vi "Transmitter_Example_Image.vi"() -> ()   [LabVIEW 2018]
uses:
  <vilib>/picture/picture.llb/imagedata.ctl
  <instrlib>/niUSRP/niUSRP Write Tx Data (CDB Cluster).vi
panel:
  out "bits":i32[](array[numeric])
  out "new picture":picture
  out "image data":T1
  in  "path to BMP file":path
  in  "Modulation parameter":T2
  out "Bits length":i32
  out "Frame Duration":dbl format="%#_6p"
  out "Waveform Graph":cluster{"t0":dbl, "dt":dbl, "Y":dbl[]}(graph)
  in  "stop":bool
  out "USRP CoercedParamters":T3={"coerced IQ rate"=100000.0, "coerced carrier frequency"=100000.0, "coerced gain"=0.0} {"coerced gain" format="%#_6f"; "coerced carrier frequency" format="%#_6p"; "coerced IQ rate" format="%#_6p"}
  out "error out":errorcluster
  in  "error in (no error)":errorcluster
  in  "USRP ControledParameters":T4={"active antenna"="TX1", "gain"=0.0, "carrier frequency"=915000000.0, "IQ rate"=1000000.0} {"IQ rate" format="%#_6p"; "carrier frequency" format="%#_6p"; "gain" format="%#_6f"}
  in  "device names":refnum<k15>="192.168.10.1"
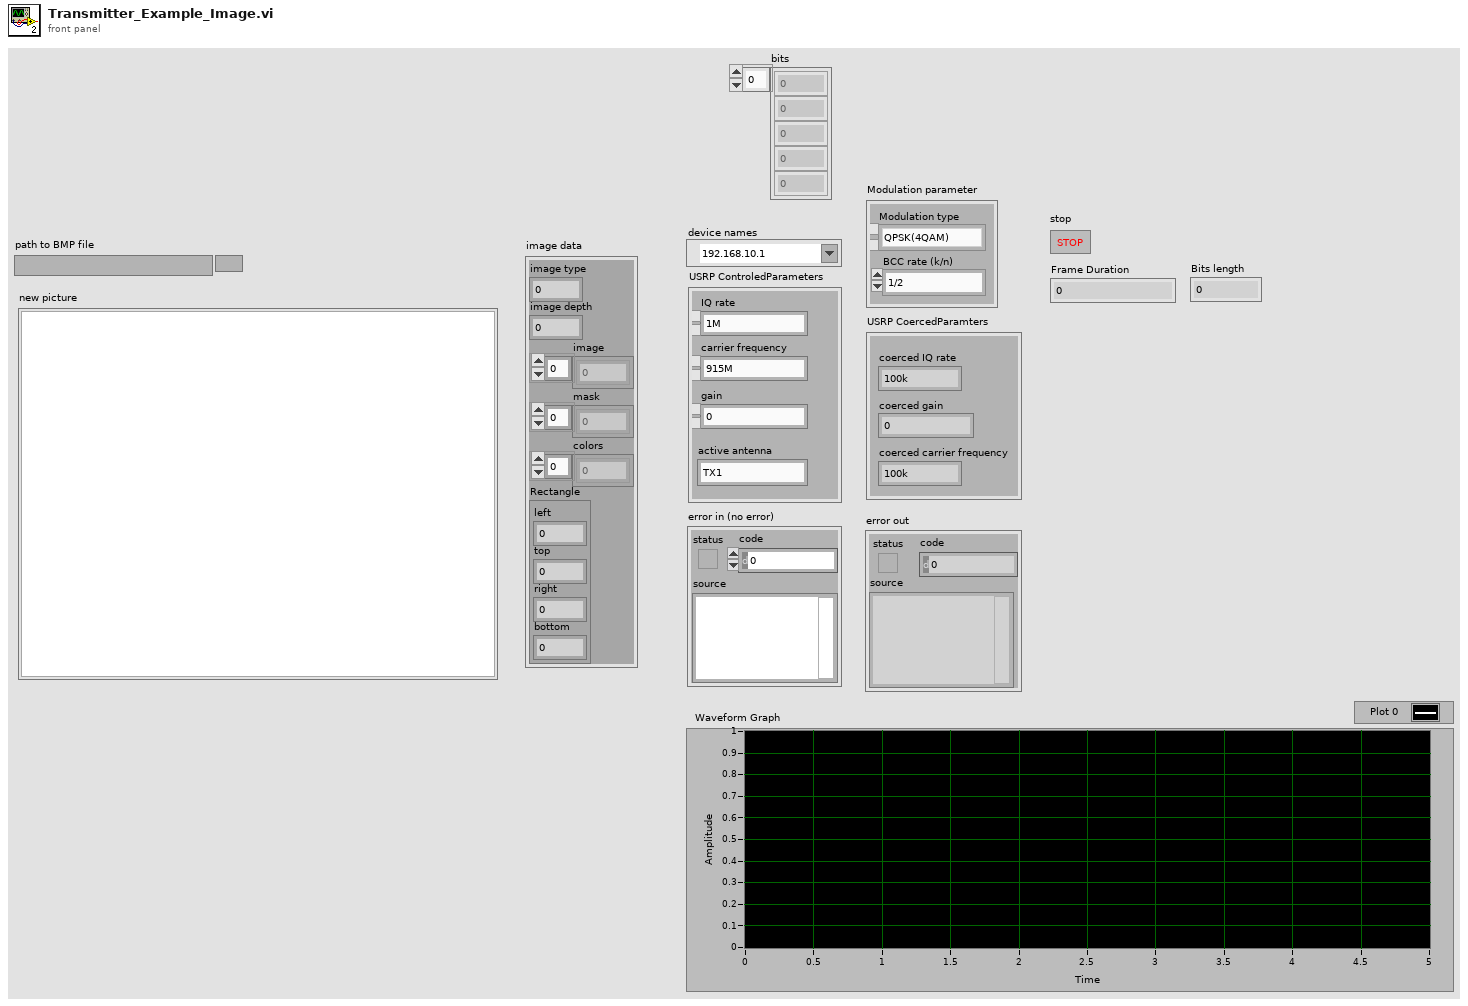
[diagram p1: front panel]
types:
  T1 = typedef "imagedata.ctl" = cluster{"image type":i32, "image depth":i32, "image":u8[], "mask":u8[], "colors":u32[], "Rectangle":cluster{"left":i16, "top":i16, "right":i16, "bottom":i16}}
  T2 = cluster{"Modulation type":enum16{"QPSK(4QAM)", "64QAM", "16QAM", "BPSK"}, "BCC rate (k/n)":enum16{"1/2", "2/3", "3/4"}}
  T3 = cluster{"coerced IQ rate":dbl, "coerced carrier frequency":dbl, "coerced gain":dbl}
  T4 = cluster{"active antenna":string, "gain":dbl, "carrier frequency":dbl, "IQ rate":dbl}
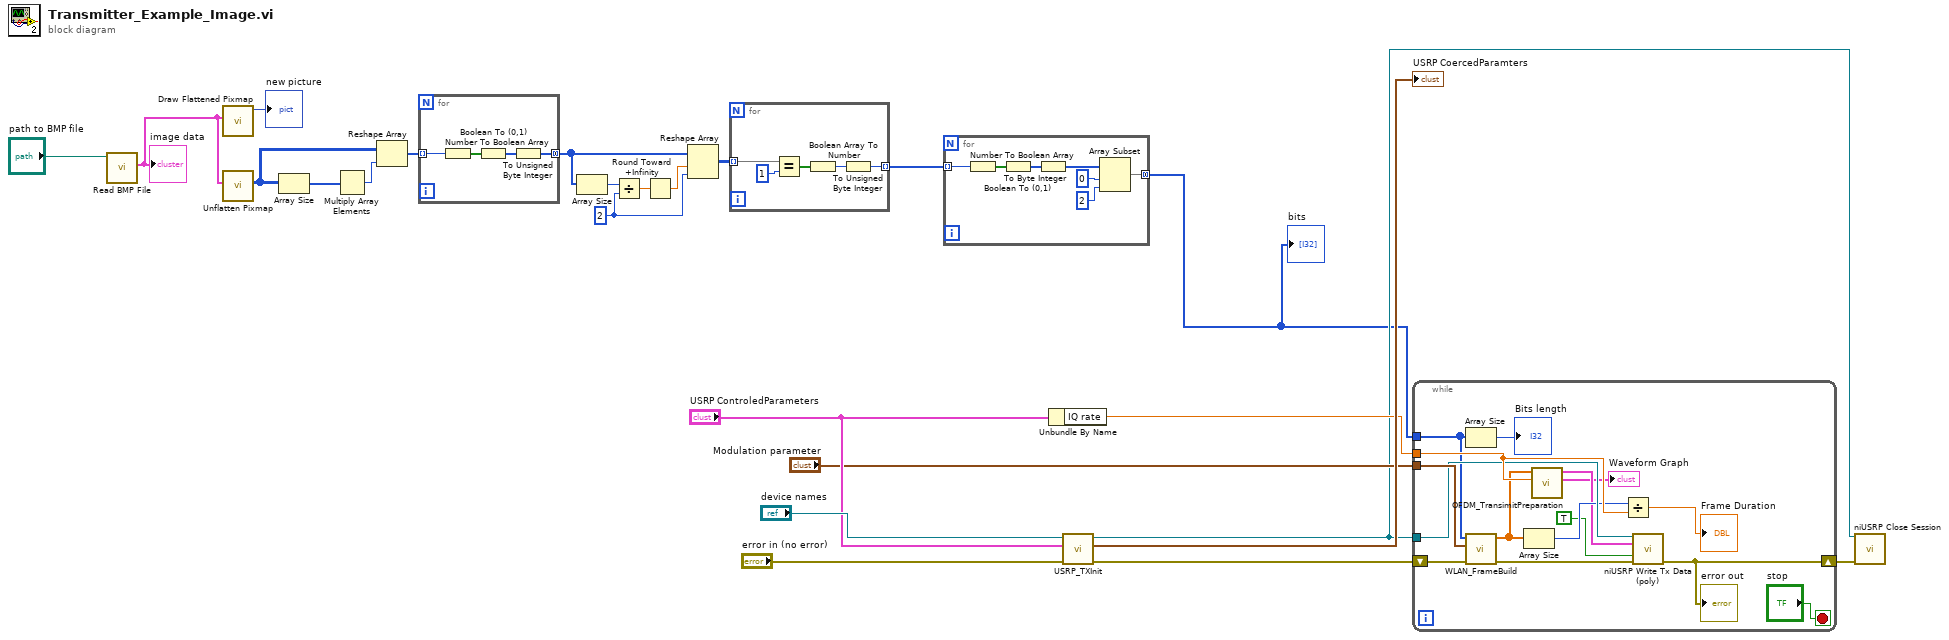
[diagram p0: block diagram]
diagram:
  w8 = 2 ("y")
  n1 = call <vilib>:"Read BMP File.vi"("path to BMP file"="path to BMP file") -> ("image data"=w13:T1)  [unwired: 8 in, 2 out]
  "image data" <- w13
  n2 = call <vilib>:"Draw Flattened Pixmap.vi"("image data"=w13) -> ("new picture"=→"new picture":picture)  [unwired: 8 in]
  n3 = call <vilib>:"Unflatten Pixmap.vi"("image data"=w13) -> ("8-bit pixmap"=w10:u8[][])  [unwired: 4 in, 6 out]
  n4 = Array Size(array=w10) -> (size(s)=w12:i32[])
  n5 = Multiply Array Elements(1:w12) -> (0:w11:i32)
  n6 = Reshape Array(w10, w11) -> (w9:u8[])
  n7 = for {
    tunnel: w9 -> [w27] mode=indexing
    tunnel: [w25] -> w4 mode=concatenating
    n8 = Number To Boolean Array(number=w27) -> (Boolean array=w28:bool[])
    n9 = Boolean To (0,1)(Boolean=w28) -> (0, 1=w26:i16[])
    n10 = To Unsigned Byte Integer(number=w26) -> (unsigned 8bit integer=w25:u8[])
  }
  n11 = Array Size(array=w4) -> (size(s)=w5:i32)
  n12 = Divide(x=w5, y=w8) -> (x/y=w6:dbl)
  n13 = Round Toward +Infinity(x=w6) -> (ceil(x): smallest int >= x=w7:dbl)
  n14 = Reshape Array(w4, w7, w8) -> (w3:u8[][])
  n15 = for {
    tunnel: w3 -> [w30] mode=indexing
    tunnel: [w29] -> w2 mode=indexing
    n16 = Equal?(x=w30, y=1) -> (x = y?=w32:bool[])
    n17 = Boolean Array To Number(Boolean array=w32) -> (number=w31:u32)
    n18 = To Unsigned Byte Integer(number=w31) -> (unsigned 8bit integer=w29:u8)
  }
  n19 = for {
    tunnel: w2 -> [w40] mode=indexing
    tunnel: [w34] -> w1 mode=concatenating
    n20 = Number To Boolean Array(number=w40) -> (Boolean array=w39:bool[])
    n21 = Boolean To (0,1)(Boolean=w39) -> (0, 1=w38:i16[])
    n22 = To Byte Integer(number=w38) -> (8bit integer=w37:i8[])
    n23 = Array Subset(array=w37, index=0, length=2) -> (w34:i8[])
  }
  "bits" <- w1
  n24 = Unbundle By Name("USRP ControledParameters") -> ("IQ rate"=w18:dbl)
  n25 = call "USRP_TXInit.vi"("device names"="device names", "USRP ControledParameters"="USRP ControledParameters", "error in (no error)"="error in (no error)") -> ("session handle out"=w17:refnum<k15>, "USRP CoercedParamters"=→"USRP CoercedParamters":T3, "error out"=w19:errorcluster)  [unwired: 5 in]
  n26 = while {
    tunnel: "Modulation parameter" -> [w55]
    tunnel: w18 -> [w53]
    tunnel: w17 -> [w52]
    tunnel: w1 -> [w50]
    shift-right: [w51] -> w16
    shift-left: w19 -> [w54]
    stop <- "stop" stop-if-true
    n27 = Array Size(array=w50) -> (size(s)=→"Bits length":i32)
    n28 = call "WLAN_FrameBuild.vi"("error in (no error)"=w54, "Modulation parameter"=w55, "data in"=w50) -> ("error out"=w45:errorcluster, "output array"=w44:cdb[])  [unwired: 4 in, 3 out]
    n29 = Array Size(array=w44) -> (size(s)=w49:i32)
    n30 = call "OFDM_TransimitPreparation.vi"("IQ rate"=w53, "array"=w44) -> ("output cluster 2"=→"Waveform Graph":cluster{"t0":dbl, "dt":dbl, "Y":cdb[]}, "output cluster"=w47:cluster{"t0":dbl, "dt":dbl, "Y":cdb[]})  [unwired: 8 in]
    n31 = Divide(x=w49, y=w53) -> (x/y=→"Frame Duration":dbl)
    n32 = call-poly <instrlib>:"niUSRP Write Tx Data (poly).vi"("session handle"=w52, "data"=w47, "end of data?"=TRUE, "error in (no error)"=w45) -> ("error out"=w51:errorcluster)  [unwired: 10 in, 1 out]
    "error out" <- w51
  }
  n33 = call <instrlib>:"niUSRP Close Session.vi"("session handle"=w17, "error in (no error)"=w16) -> ()  [unwired: 13 in, 1 out]
